vi "Dashboard Main.vi"() -> ()   [LabVIEW 2012]
uses:
  <vilib>/event_ctls.llb/eventvkey.ctl
  <vilib>/Utility/miscctls.llb/LVPointTypeDef.ctl
  <vilib>/Utility/config.llb/Read Key (String).vi
  <vilib>/Utility/config.llb/Read Key (I32).vi
  <vilib>/Utility/config.llb/Write Key (String).vi
  <vilib>/Utility/config.llb/Write Key (I32).vi
  <vilib>/Utility/config.llb/NI_LVConfig.lvlib
panel:
  in  "Camera Settings":T1={"Frate Rate"=30, "Compression"=70, "Size"=1} {"Frate Rate" scale=1.0..30.0; "Size" items=["640x480", "320x240", "160x120"]}
  out "Mode":T2(ring)=enum.""
  out "Camera IP":string="0.0.0.11"
  in  "Dashboard Tab":T3(tab)=enum."Drive Info"
  out "GO!! GO!! GO!!":bool
  out "Angle Ready":bool
  out "Shooter Speed":T4(ring)
  out "Shooter Encoder\nDead!!":bool
  out "Speed Ready":bool
  out "Dashboard Code Verzion":string
  out "Robot Code Version":string
  out "Display Loop speed (Hz)":dbl
  out "Shooter Angle":T5(ring)
  out "Shooter Good":bool
  out "Shooter Speed":dbl(graph)
  out "Wheel Speed":dbl
  out "Shooter Output":dbl
  out "Shooter Speed":T4(ring)
  out "Encoder Angle":dbl
  out "Debug Mode":bool
  out "Left Encoder":dbl
  out "Right Encoder":dbl
  out "Encoder Average":dbl
  out "Left Encoder Rate":dbl
  out "Right Encoder Rate":dbl
  out "Encoder Average Rate":dbl
  out "Gyro":dbl
  out "Battery Value":dbl(slide) scale=0.0..14.0 scale format="%#_2e"
  out "Battery":sgl(graph)
  out "JS1 Z":dbl(slide) scale=-1.0..1.0 scale format="%#_2e"
  out "JS2 Z":dbl(slide) scale=-1.0..1.0 scale format="%#_2e"
  out "Joystick 1":cluster{"X":dbl, "Y":dbl}[](graph)
  out "Joystick 2":cluster{"X":dbl, "Y":dbl}[](graph)
  out "JS Buttons 1":T6
  out "JS Buttons 2":T6
  out "MotorSlide4":dbl(slide) scale=-1.0..1.0 scale format="%#_2e"
  out "MotorSlide3":dbl(slide) scale=-1.0..1.0 scale format="%#_2e"
  out "MotorSlide2":dbl(slide) scale=-1.0..1.0 scale format="%#_2e"
  in  "MotorName3":string="Front Left"
  in  "MotorName4":string="Front Right"
  in  "MotorName1":string="Rear Left"
  in  "MotorName2":string="Rear Right"
  out "MotorChart4":dbl(graph)
  out "MotorChart3":dbl(graph)
  out "MotorChart2":dbl(graph)
  out "MotorSlide1":dbl(slide) scale=-1.0..1.0 scale format="%#_2e"
  out "MotorChart1":dbl(graph)
  out "Robot IP":string="0.0.0.0"
  in  "Debug Mode":bool
  in  "Slider":dbl(slide) scale=0.0..100.0 scale format="%#_3g"
  in  "On/Off":bool caption="Solenoid"
  in  "Test Name":u16(ring) items=["Select the test to run...", "Example Test", "-------------------------------", "List of tests is built in robot code.", "Replace with your own automated tests."]
  in  "Test Tree":string(tree)
  in  "Motor":cluster{"Value":dbl, "Enable":bool} {"Value" scale=-1.0..1.0 scale format="%#_3g"}
  out "Progress":T7 {"Test Progress" scale=0.0..100.0}
  in  "Rev/Fwd":cluster{"Forward":bool, "Reverse":bool}
  in  "Ring":u16(ring) items=["Auto", "Fixed indoor", "Fixed outdoor 1", "Fixed outdoor 2", "Fixed fluorescent 1", "Fixed fluorescent 2", "Hold current"]
  in  "Listbox":i32(listbox)
  in  "Viewer":T8(tab)
  in  "Enable Processing":bool
  out "Mbps":dbl format="%#.1g"
  in  "Enable":bool=TRUE
  in  "DB Camera Config":bool
  out "Mbps":bool
  out "fps":dbl format="%#.1g"
  out "Image Error Message":string="Timeout in Camera Communications"
  out "Camera Image":T9(plugin-control)
  out "Vision Angle":dbl
  out "Buttons 1":cluster{"1":bool, "2":bool, "3":bool}
  out "Kinect 1":cluster{"X":dbl, "Y":dbl, "Z":dbl} {"X" scale=1.0..-1.0; "Y" scale=1.0..-1.0; "Z" scale=1.0..-1.0}
  out "Buttons 2":cluster{"1":bool, "2":bool, "3":bool}
  out "Kinect 2":cluster{"X":dbl, "Y":dbl, "Z":dbl} {"X" scale=1.0..-1.0; "Y" scale=1.0..-1.0; "Z" scale=1.0..-1.0}
  out "Version":string
  out "Skeleton Picture":picture
  out "Players":i8
  out "Tree":string(tree)
  # "Drive & Motors"
  # "Robot IP:"
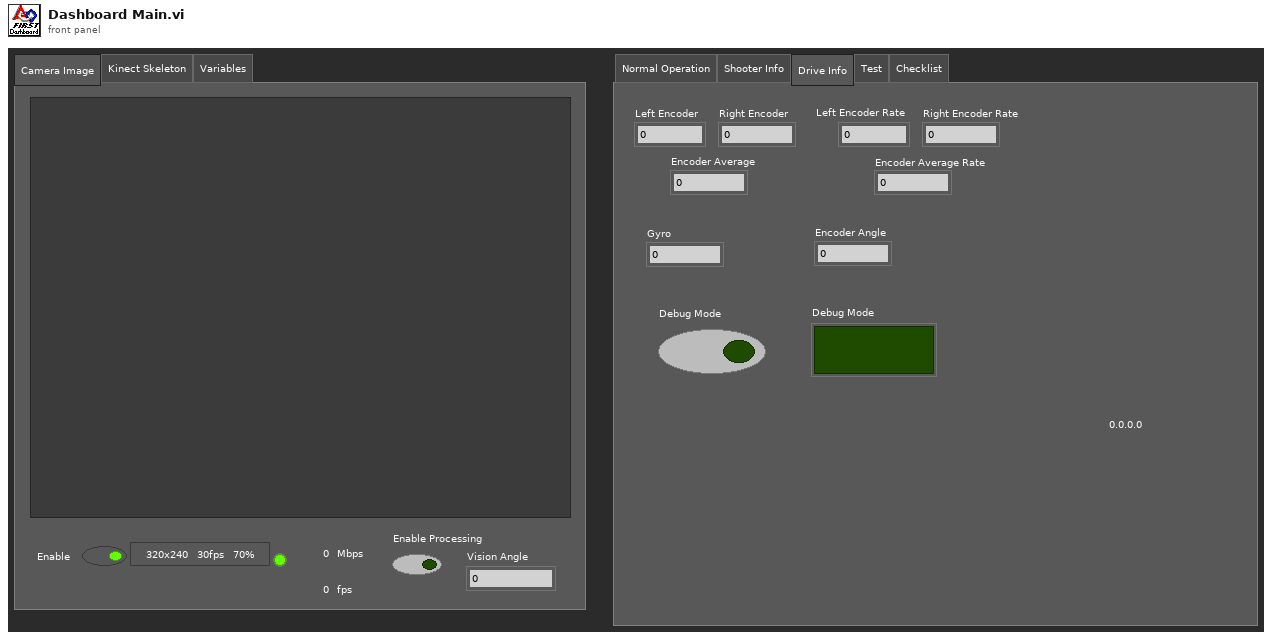
[diagram p1: front panel]
types:
  T1 = cluster{"Frate Rate":i32, "Compression":i32, "Size":u16}
  T2 = enum8{"Tele-Op Disabled", "Tele-Op Enabled", "Auto Disabled", "Auto Enabled", "Test Disabled", "Test Enabled", ""}
  T3 = enum32{"Normal Operation", "Shooter Info", "Drive Info", "Test", "Checklist"}
  T4 = enum16{"Off", "Close Pyramid 3pt", "Far Pyramid 3pt", "Feeder Shot", "UD Far 3pt Shot"}
  T5 = enum16{"Close 3pt Shot", "Far 3pt Shot", "Feeding"}
  T6 = cluster{bool, bool, bool, bool, bool, bool, bool, bool, bool, bool, bool, bool}
  T7 = cluster{"Test Progress":u8, "Test Progress Text":string}
  T8 = enum32{"Camera Image", "Kinect Skeleton", "Variables"}
  T9 = typedef "IMAQ Image.ctl" = refnum<image>
  T10 = typedef "Image Type" = u32
  T11 = cluster{"Competition mode":bool, "Robot Link":bool, "Autonomous":bool, "Enabled":bool, "E-Stop":bool, "Simulated":bool, "TestMode":bool, "Docked Window":bool}
  T12 = cluster{"Boolean Array[0]":bool, "Boolean Array[1]":bool, "Boolean Array[2]":bool, "Boolean Array[3]":bool, "Boolean Array[4]":bool, "Boolean Array[5]":bool, "Boolean Array[6]":bool, "Boolean Array[7]":bool, "Boolean Array[8]":bool, "Boolean Array[9]":bool, "Boolean Array[10]":bool, "Boolean Array[11]":bool}
  T13 = typedef "LVPointTypeDef.ctl" = cluster{"Horizontal":i16, "Vertical":i16}
  T14 = typedef "LVRectTypeDef.ctl" = cluster{"Left":i16, "Top":i16, "Right":i16, "Bottom":i16}
  T15 = typedef "LVBoundsTypeDef.ctl" = cluster{"Width":u32, "Height":u32}
  T16 = typedef "SkeletonTrackState.ctl" = enum32{"NotTracked", "PositionOnly", "Tracked"}
  T17 = cluster{"TrackingState":u8[], "Position":cluster{"x":sgl, "y":sgl, "z":sgl}, cluster{"x":sgl, "y":sgl, "z":sgl, sgl}[], "TrackState":T16}
  T18 = cluster{cluster{"ScaledToPercentRange":dbl, "ScaledToPercentRange":dbl, "ScaledToPercentRange":dbl}, cluster{bool, bool, bool}}[]
  T19 = cluster{cluster{"ScaledToPercentRange":dbl, "ScaledToPercentRange":dbl, "ScaledToPercentRange":dbl}, cluster{bool, bool, bool}}
  T20 = cluster{"ScaledToPercentRange":dbl, "ScaledToPercentRange":dbl, "ScaledToPercentRange":dbl}
  T21 = typedef "NI_LVConfig.lvlib/Config Data RefNum.ctl" = refnum<k1>
  T22 = typedef "eventvkey.ctl" = enum16{"ASCII", "Enter", "Return", "Shift", "Ctrl", "Alt", "Cmd", "Opt", "Caps", "NumLock", "Clear", "Break", "Up", "Down", "Left", "Right", "Insert", "Delete", "Home", "End", "PageUp", "PageDown", "Escape", "Help", "Pause", "ScrollLock", "F1", "F2", "F3", "F4", "F5", "F6", "F7", "F8", "F9", "F10", "F11", "F12", "F13", "F14", "F15", "F16", "F17", "F18", "F19", "F20", "F21", "F22", "F23", "F24", "Play", "VolumeUp", "VolumeDown", "Mute", "Two Byte Char"}
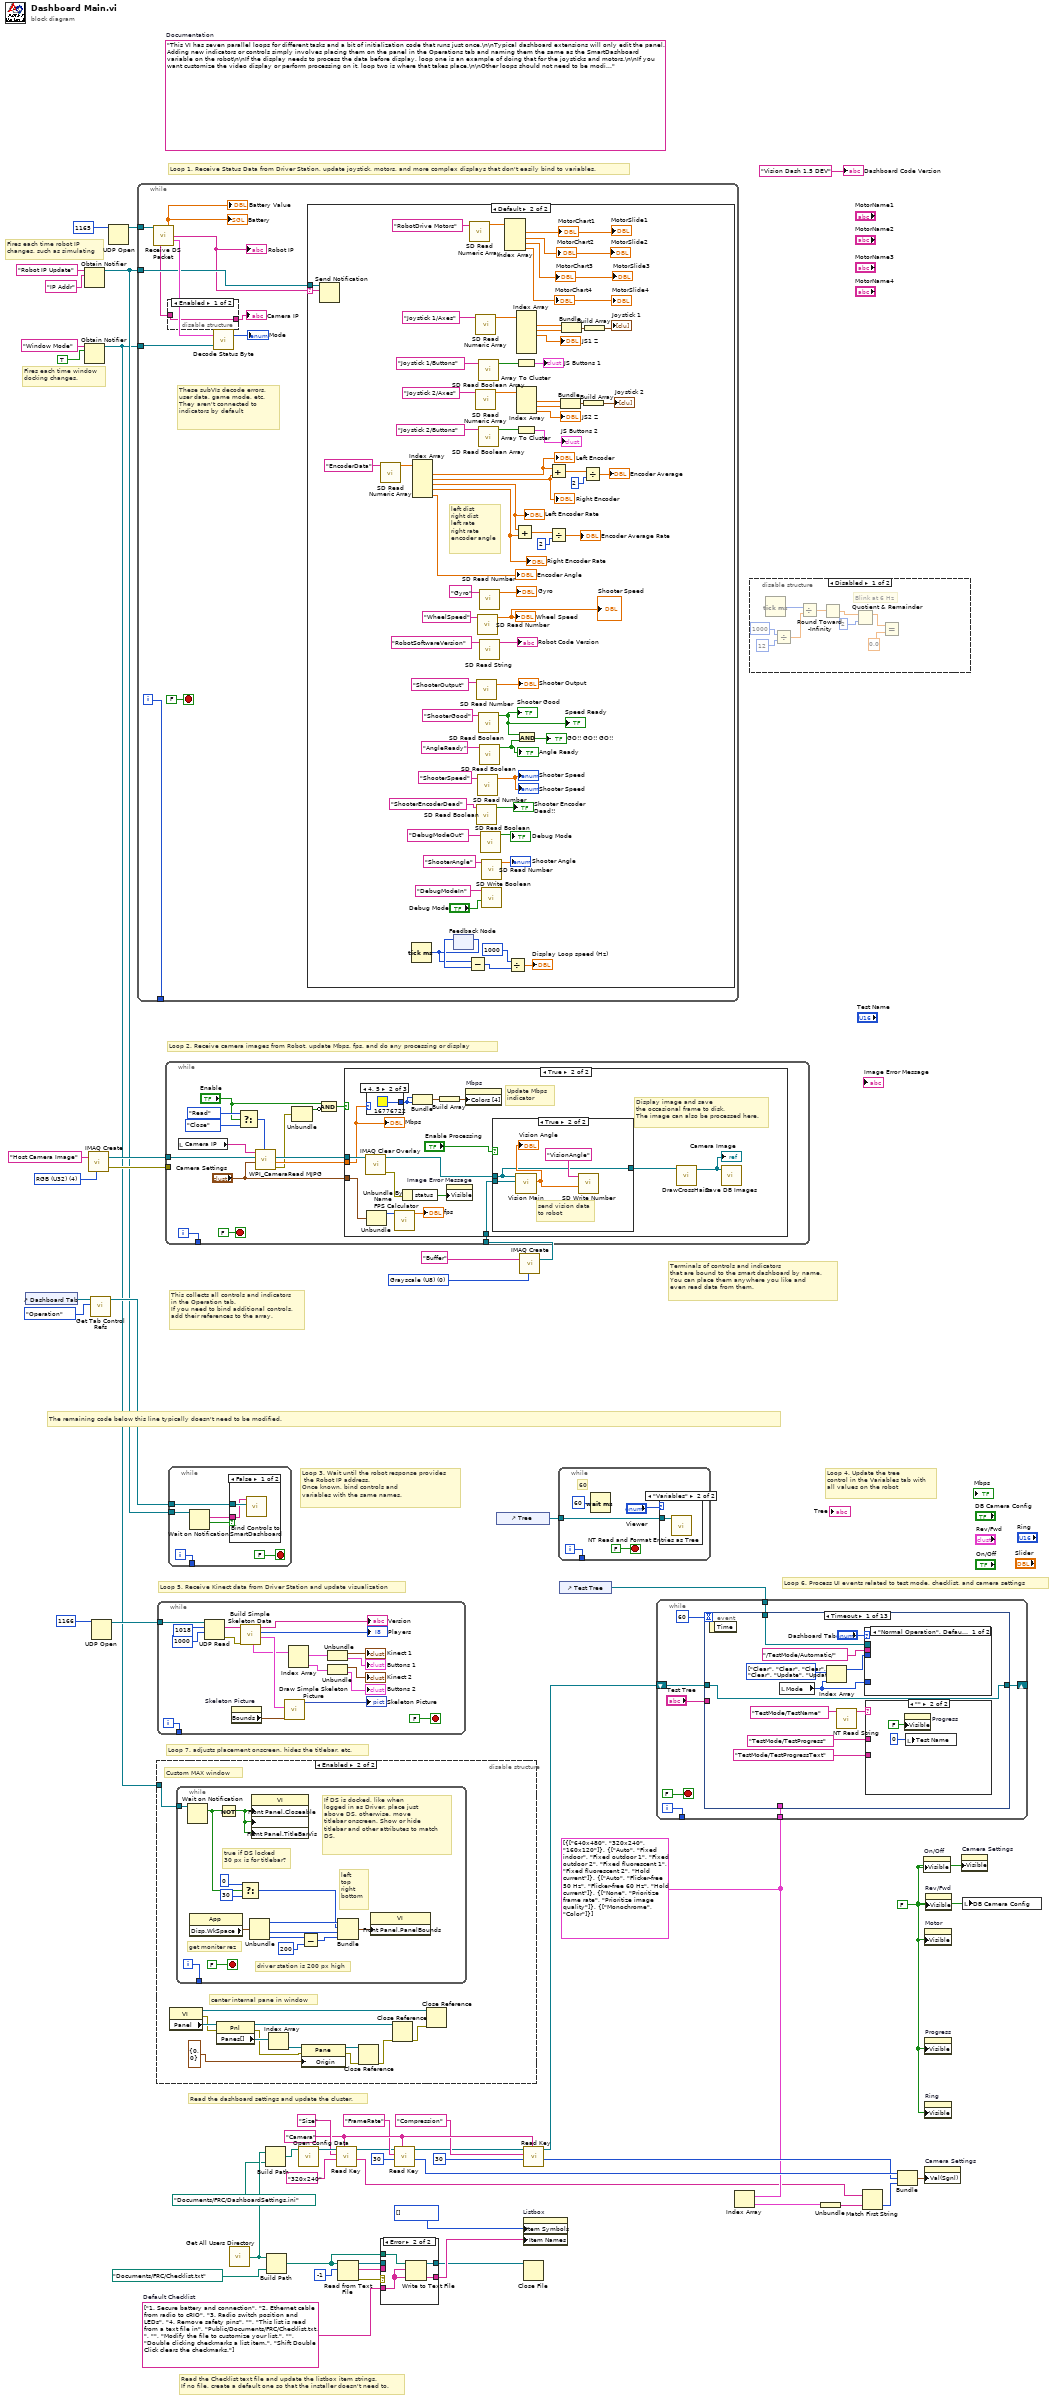
[diagram p0: block diagram]
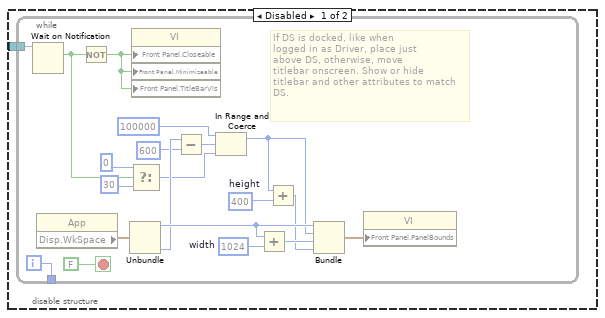
[diagram p3: hidden frame]
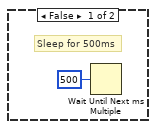
[diagram p5: hidden frame]
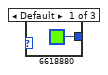
[diagram p7: hidden frame]
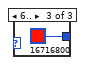
[diagram p8: hidden frame]
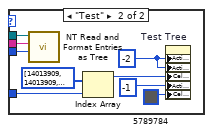
[diagram p10: hidden frame]
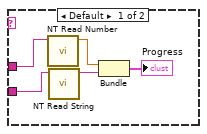
[diagram p11: hidden frame]
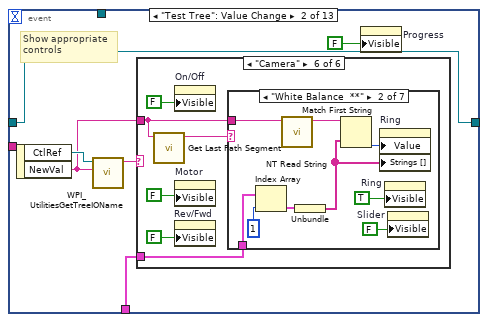
[diagram p12: hidden frame]
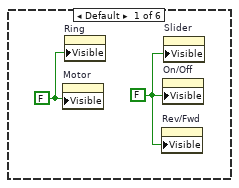
[diagram p13: hidden frame]
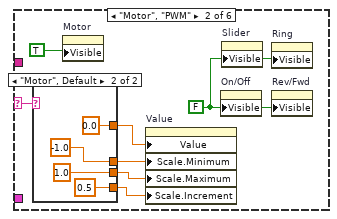
[diagram p14: hidden frame]
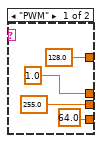
[diagram p15: hidden frame]
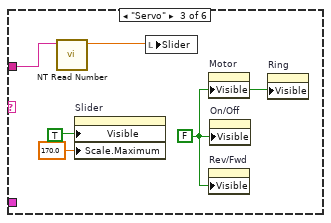
[diagram p16: hidden frame]
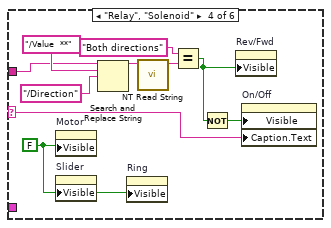
[diagram p17: hidden frame]
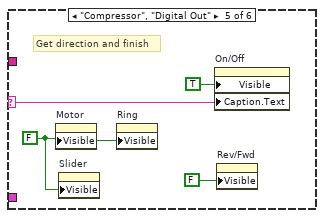
[diagram p18: hidden frame]
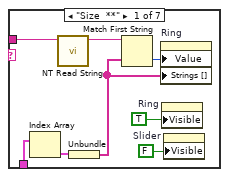
[diagram p19: hidden frame]
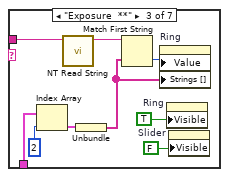
[diagram p20: hidden frame]
diagram:
  w3 = T10 0 items=["Grayscale (U8)", "Grayscale (I16)", "Grayscale (SGL)", "Complex (CSG)", "RGB (U32)", "HSL (U32)", "RGB (U64)", "Grayscale (U16)"] ("Image Type")
  w25 = "Camera"
  w17 = cluster{string[]}[] [{["640x480", "320x240", "160x120"]}, {["Auto", "Fixed indoor", "Fixed outdoor 1", "Fixed outdoor 2", "Fixed fluorescent 1", "Fixed fluorescent 2", "Hold current"]}, {["Auto", "Flicker-free 50 Hz", "Flicker-free 60 Hz", "Hold current"]}, {["None", "Prioritize frame rate", "Prioritize image quality"]}, {["Monochrome", "Color"]}]
  w33 = string[] ["1. Secure battery and connection", "2. Ethernet cable from radio to cRIO", "3. Radio switch position and LEDs", "4. Remove safety pins", "", "This list is read from a text file in", "Public/Documents/FRC/Checklist.txt.", "", "Modify the file to customize your list.", "", "Double clicking checkmarks a list item.", "Shift Double Click clears the checkmarks."]  # Default Checklist
  w31 = FALSE ("Visible")
  (unwired) "This VI has seven parallel loops for different tasks and a bit of initialization code that runs just once.\n\nTypical dashboard extensions will only edit the panel. Adding new indicators or controls simply involves placing them on the panel in the Operations tab and naming them the same as the SmartDashboard variable on the robot\n\nIf the display needs to process the data before display, loop one is an example of doing that for the joysticks and motors.\n\nIf you want customize the video display or perform processing on it, loop two is where that takes place.\n\nOther loops should not need to be modified. They are pretty standard, and document the task they perform."  # Documentation
  w54 = T10 4 items=["Grayscale (U8)", "Grayscale (I16)", "Grayscale (SGL)", "Complex (CSG)", "RGB (U32)", "HSL (U32)", "RGB (U64)"] ("Image Type")
  # "Fires each time robot IP\nchanges, such as simulating"
  # "Fires each time window\ndocking changes."
  # "Read the Checklist text file and update the listbox item strings.\nIf no file, create a default one so that the installer doesn't need to."
  # "This collects all controls and indicators\nin the Operation tab.\nIf you need to bind additional controls,\nadd their references to the array."
  # "The remaining code below this line typically doesn't need to be modified."
  # "Loop 6. Process UI events related to test mode, checklist, and camera settings"
  # "Read the dashboard settings and update the cluster."
  # "Terminals of controls and indicators\nthat are bound to the smart dashboard by name.\nYou can place them anywhere you like and\neven read data from them."
  # "Loop 4. Update the tree\ncontrol in the Variables tab with\nall values on the robot"
  # "Loop 3. Wait until the robot response provides\n the Robot IP address.\nOnce known, bind controls and\nvariables with the same names."
  # "Loop 5. Receive Kinect data from Driver Station and update visualization"
  # "Loop 7. adjusts placement onscreen, hides the titlebar, etc."
  # "Loop 1. Receive Status Data from Driver Station, update joystick, motors, and more complex displays that don't easily bind to variables."
  # "Loop 2. Receive camera images from Robot, update Mbps, fps, and do any processing or display"
  n1 = control-ref of="Dashboard Tab"() -> (w47:refnum<vi>)
  n2 = Obtain Notifier(name (unnamed)="Robot IP Update", notification data type="IP Addr" ("name (unnamed)")) -> (notifier out=w44:refnum<notifier>)  [unwired: 2 in, 2 out]
  n3 = Obtain Notifier(name (unnamed)="Window Mode", notification data type=TRUE) -> (notifier out=w37:refnum<notifier>)  [unwired: 2 in, 2 out]
  n4 = call "IMAQ Create"("Image Name"="Host Camera Image", "Image Type"=w54) -> ("New Image"=w52:T9, "error out"=w51:errorcluster)  [unwired: 2 in, 1 out]
  n5 = call <vilib>:"Get Tab Control Refs.vi"("Page Index"=enum32{"Operation", "Test"}."Operation" ("Dashboard Tab"), "TabControl in"=w47) -> ("ControlsOnPage"=w48:refnum<vi>[])  [unwired: 9 in]
  n6 = UDP Open(11:u16 1166 ("port")) -> (port=w49:refnum<k16>)  [unwired: 2 in, 4 out]
  n7 = UDP Open(11:u16 1165 ("port")) -> (port=w55:refnum<k16>)  [unwired: 2 in, 4 out]
  n8 = while {
    tunnel: w55 -> [w65]
    tunnel: w44 -> [w60]
    tunnel: w37 -> [w63]
    tunnel: [w61] -> _
    i -> [w61]
    stop <- FALSE stop-if-true
    # "These subVIs decode errors, user data, game mode, etc.\nThey aren't connected to indicators by default"
    n9 = call "Receive DS Packet.vi"("Recv Socket"=w65) -> ("Battery"=→"Battery" →"Battery Value":sgl, "Robot IP Address"=w59:string, "Status"=w66:T11, "Camera IP Address"=w57:string)  [unwired: 1 in, 10 out]
    "Robot IP" <- w59
    n10 = disable-structure shown="Enabled" {
      disable-tunnel: [w68 "10.16.76.11" ("Camera IP")] -> w58
      disable-tunnel: w57 -> [w68 _]
      frame Enabled {
      }
      frame Disabled {
      }
    }
    "Camera IP" <- w58
    n11 = call "Decode Status Byte.vi"("Window Mode Notifier"=w63, "Status"=w66) -> ("Mode"=→"Mode":T2)  [unwired: 1 out]
    n12 = case shown="Default" w59 {
      selector: w59 -> [_ w111]
      tunnel: w60 -> [_ w112]
      frame "0.0.0.0" {
        # "Robot not responding, don't poll the variables"
      }
      frame Default {
        # "left dist\nright dist\nleft rate\nright rate\nencoder angle"
        n13 = Send Notification(notification=w111, notifier=w112) -> ()  [unwired: 1 in, 2 out]
        n14 = call <vilib>:"SD Read Numeric Array.vi"("Name"="EncoderData") -> ("Numeric Array"=w98:dbl[])  [unwired: 8 in, 2 out]
        n15 = Tick Count (ms)() -> (millisecond timer value=w80:u32)
        n16 = Index Array(array=w98) -> (element #1=w97:dbl, element #2=w96:dbl, element #3=w92:dbl, element #4=w91:dbl, element #5=→"Encoder Angle":dbl)  [unwired: 5 in]
        "Left Encoder" <- w97
        "Right Encoder" <- w96
        "Left Encoder Rate" <- w92
        "Right Encoder Rate" <- w91
        n17 = feedback-in #1(w80) -> ()
        n18 = feedback #1() -> (w81:u32)  [unwired: 1 in]
        n19 = Subtract(x=w80, y=w81) -> (x-y=w79:u32)
        n20 = call <vilib>:"SD Read Numeric Array.vi"("Name"="RobotDrive Motors") -> ("Numeric Array"=w135:dbl[])  [unwired: 8 in, 2 out]
        n21 = call <vilib>:"SD Read Numeric Array.vi"("Name"="Joystick 1/Axes") -> ("Numeric Array"=w128:dbl[])  [unwired: 8 in, 2 out]
        n22 = call <vilib>:"SD Read Numeric Array.vi"("Name"="Joystick 2/Axes") -> ("Numeric Array"=w122:dbl[])  [unwired: 8 in, 2 out]
        n23 = call <vilib>:"SD Read Number.vi"("Name"="ShooterOutput") -> ("Numeric"=→"Shooter Output":dbl)  [unwired: 8 in, 2 out]
        n24 = call <vilib>:"SD Read Boolean.vi"("Name"="ShooterEncoderDead") -> ("Boolean"=→"Shooter Encoder\nDead!!":bool)  [unwired: 8 in, 2 out]
        n25 = call <vilib>:"SD Read Number.vi"("Name"="ShooterSpeed") -> ("Numeric"=→"Shooter Speed" →"Shooter Speed":dbl)  [unwired: 8 in, 2 out]
        n26 = call <vilib>:"SD Read Number.vi"("Name"="WheelSpeed") -> ("Numeric"=→"Wheel Speed" →"Shooter Speed":dbl)  [unwired: 8 in, 2 out]
        n27 = call <vilib>:"SD Read Boolean Array.vi"("Name"="Joystick 1/Buttons") -> ("Boolean Array"=w130:bool[])  [unwired: 8 in, 2 out]
        n28 = call <vilib>:"SD Read Boolean Array.vi"("Name"="Joystick 2/Buttons") -> ("Boolean Array"=w121:bool[])  [unwired: 8 in, 2 out]
        n29 = call <vilib>:"SD Read Boolean.vi"("Name"="ShooterGood") -> ("Boolean"=w85:bool)  [unwired: 8 in, 2 out]
        "Shooter Good" <- w85
        "Speed Ready" <- w85
        n30 = call <vilib>:"SD Read Number.vi"("Name"="Gyro") -> ("Numeric"=→"Gyro":dbl)  [unwired: 8 in, 2 out]
        n31 = call <vilib>:"SD Read String.vi"("Name"="RobotSoftwareVersion") -> ("String"=→"Robot Code Version":string)  [unwired: 8 in, 2 out]
        n32 = call <vilib>:"SD Read Boolean.vi"("Name"="AngleReady") -> ("Boolean"=w84:bool)  [unwired: 8 in, 2 out]
        "Angle Ready" <- w84
        n33 = call <vilib>:"SD Read Boolean.vi"("Name"="DebugModeOut") -> ("Boolean"=→"Debug Mode":bool)  [unwired: 8 in, 2 out]
        n34 = call <vilib>:"SD Read Number.vi"("Name"="ShooterAngle") -> ("Numeric"=→"Shooter Angle":dbl)  [unwired: 8 in, 2 out]
        n35 = call <vilib>:"SD Write Boolean.vi"("Boolean"="Debug Mode", "Name"="DebugModeIn") -> ()  [unwired: 8 in, 2 out]
        n36 = Index Array(array=w135) -> (element #1=→"MotorChart1" →"MotorSlide1":dbl, element #2=→"MotorSlide2" →"MotorChart2":dbl, element #3=→"MotorChart3" →"MotorSlide3":dbl, element #4=→"MotorChart4" →"MotorSlide4":dbl)  [unwired: 4 in]
        n37 = Divide(x=1000, y=w79) -> (x/y=→"Display Loop speed (Hz)":dbl)
        n38 = Add(x=w92, y=w91) -> (x+y=w93:dbl)
        n39 = Array To Cluster(array=w130) -> (cluster=→"JS Buttons 1":T12)
        n40 = Array To Cluster(array=w121) -> (cluster=→"JS Buttons 2":T12)
        n41 = Index Array(array=w128) -> (element #1=w125:dbl, element #2=w126:dbl, element #3=→"JS1 Z":dbl)  [unwired: 6 in, 3 out]
        n42 = Index Array(array=w122) -> (element #1=w117:dbl, element #2=w116:dbl, element #3=→"JS2 Z":dbl)  [unwired: 3 in]
        n43 = And(x=w85, y=w84) -> (x .and. y?=→"GO!! GO!! GO!!":bool)
        n44 = Add(x=w97, y=w96) -> (x+y=w107:dbl)
        n45 = Divide(x=w93, y=2) -> (x/y=→"Encoder Average Rate":dbl)
        n46 = Bundle("Numeric"=w117, "Numeric"=w116) -> (w118:cluster{"Numeric":dbl, "Numeric":dbl})  [unwired: 1 in]
        n47 = Bundle("Numeric"=w125, "Numeric"=w126) -> (w124:cluster{"Numeric":dbl, "Numeric":dbl})  [unwired: 1 in]
        n48 = Divide(x=w107, y=2) -> (x/y=→"Encoder Average":dbl)
        n49 = Build Array(w118) -> (→"Joystick 2":cluster{"Numeric":dbl, "Numeric":dbl}[])
        n50 = Build Array(w124) -> (→"Joystick 1":cluster{"Numeric":dbl, "Numeric":dbl}[])
      }
    }
  }
  n51 = disable-structure shown="Enabled" {
    disable-tunnel: w37 -> [w139 w172]
    frame Disabled {
      n52 = while {
        tunnel: w139 -> [w158]
        tunnel: [w156] -> _
        i -> [w156]
        stop <- FALSE stop-if-true
        w148 = 1024  # width
        w151 = 400  # height
        # "If DS is docked, like when\nlogged in as Driver, place just\nabove DS, otherwise, move\ntitlebar onscreen. Show or hide\ntitlebar and other attributes to match\nDS."
        n53 = Wait on Notification(notifier=w158) -> (notification=w143:bool)  [unwired: 3 in, 3 out]
        n54 = property class="App"() -> ("Disp.WkSpace"=w154:T14)  [unwired: 2 in, 2 out]
        n55 = Not(x=w143) -> (.not. x?=w157:bool)
        n56 = Unbundle(w154) -> ("Left"=w152:i16, "Bottom"=w149:i16)  [unwired: 2 out]
        n57 = Select(t=0, s=w143, f=30) -> (s? t:f=w142:i32)
        n58 = property class="VI"("Front Panel.Closeable"=w157, "Front Panel.Minimizeable"=w157, "Front Panel.TitleBarVis"=w157) -> ()  [unwired: 2 in, 2 out]
        n59 = Subtract(x=w149, y=600) -> (x-y=w146:i32)
        n60 = In Range and Coerce(upper limit=100000, x=w146, lower limit=w142) -> (coerced(x)=w140:i32)  [unwired: 1 out]
        n61 = Add(x=w152, y=w148) -> (x+y=w153:i32)
        n62 = Add(x=w140, y=w151) -> (x+y=w150:i32)
        n63 = Bundle("Left"=w152, w140, w153, w150) -> (w155:cluster{"Left":i16, i32, i32, i32})  [unwired: 1 out]
        n64 = property class="VI"("Front Panel.PanelBounds"=w155) -> ()  [unwired: 2 in, 2 out]
      }
    }
    frame Enabled {
      # "center internal pane in window"
      # "Custom MAX window"
      n65 = property class="VI"() -> (reference out=w165:refnum<vi>, error out=w164:errorcluster, "Panel"=w171:refnum<vi>)  [unwired: 2 in]
      n66 = while {
        tunnel: w172 -> [w186]
        tunnel: [w184] -> _
        i -> [w184]
        stop <- FALSE stop-if-true
        # "driver station is 200 px high"
        # "true if DS locked\n30 px is for titlebar?"
        # "left\ntop\nright\nbottom"
        # "get moniter rez"
        # "If DS is docked, like when\nlogged in as Driver, place just\nabove DS, otherwise, move\ntitlebar onscreen. Show or hide\ntitlebar and other attributes to match\nDS."
        n67 = Wait on Notification(notifier=w186) -> (notification=w178:bool)  [unwired: 3 in, 3 out]
        n68 = property class="App"() -> ("Disp.WkSpace"=w182:T14)  [unwired: 2 in, 2 out]
        n69 = Not(x=w178) -> (.not. x?=w185:bool)
        n70 = Select(t=0, s=w178, f=30) -> (s? t:f=w176:i32)
        n71 = Unbundle(w182) -> ("Left"=w181:i16, "Right"=w177:i16, "Bottom"=w174:i16)  [unwired: 1 out]
        n72 = property class="VI"("Front Panel.Closeable"=w185, "Front Panel.Minimizeable"=w185, "Front Panel.TitleBarVis"=w185) -> ()  [unwired: 2 in, 2 out]
        n73 = Subtract(x=w174, y=i16 200) -> (x-y=w175:i16)
        n74 = Bundle("Left"=w181, w176, "Right"=w177, w175) -> (w183:cluster{"Left":i16, i32, "Right":i16, i16})  [unwired: 1 out]
        n75 = property class="VI"("Front Panel.PanelBounds"=w183) -> ()  [unwired: 2 in, 2 out]
      }
      n76 = property class="Pnl"(reference=w171, error in=w164) -> (reference out=w166:refnum<vi>, error out=w163:errorcluster, "Panes[]"=w170:refnum<vi>[])
      n77 = Index Array(array=w170) -> (element=w169:refnum<vi>)  [unwired: 1 in]
      n78 = property class="Pane"(reference=w169, error in=w163, "Origin"=T13 {"Horizontal"=0, "Vertical"=0}) -> (reference out=w167:refnum<vi>, error out=w162:errorcluster)
      n79 = Close Reference(reference=w167, error in (no error)=w162) -> (error out=w161:errorcluster)
      n80 = Close Reference(reference=w166, error in (no error)=w161) -> (error out=w160:errorcluster)
      n81 = Close Reference(reference=w165, error in (no error)=w160) -> ()  [unwired: 1 out]
    }
  }
  n82 = while {
    tunnel: w49 -> [w204]
    tunnel: [w189] -> _
    i -> [w189]
    stop <- FALSE stop-if-true
    n83 = UDP Read(connection ID=w204, max size (548)=1018 ("bytes to read"), timeout ms (25000)=1000) -> (data out=w198:string, error out=w188:errorcluster)  [unwired: 1 in, 3 out]
    n84 = property on="Skeleton Picture" class="Pict"() -> ("Bounds"=w200:T15)  [unwired: 2 in, 2 out]
    n85 = call "Build Simple Skeleton Data.vi"("error in (no error)"=w188, "data in"=w198) -> ("Skeleton Data"=w199:T17, "NumPlayers"=→"Players":i8, "Version String"=→"Version":string, "Simple Joystick Info"=w196:T18)  [unwired: 5 in, 1 out]
    n86 = call "Draw Simple Skeleton Picture.vi"("Bounds"=w200, "Simple Skeleton"=w199) -> ("new picture out"=→"Skeleton Picture":picture)  [unwired: 9 in]
    n87 = Index Array(array=w196) -> (element #1=w195:T19, element #2=w194:T19)  [unwired: 2 in]
    n88 = Unbundle(w195) -> (→"Kinect 1":T20, →"Buttons 1":cluster{bool, bool, bool})
    n89 = Unbundle(w194) -> (→"Kinect 2":T20, →"Buttons 2":cluster{bool, bool, bool})
  }
  n90 = while {
    tunnel: w48 -> [w212]
    tunnel: w44 -> [w209]
    tunnel: [w207] -> _
    i -> [w207]
    stop <- FALSE stop-if-true
    n91 = Wait on Notification(notifier=w209) -> (notification=w208:string, timed out?=w210:bool)  [unwired: 3 in, 2 out]
    n92 = case shown="False" w210 {
      tunnel: w212 -> [w214 _]
      tunnel: w208 -> [w213 _]
      frame False {
        n93 = call <vilib>:"Bind Controls to SmartDashboard.vi"("Bound Control Refs"=w214, "Server IP Address"=w213) -> ()  [unwired: 10 in]
      }
      frame True {
      }
    }
  }
  n94 = call "Get All Users Directory.vi"() -> ("All User Path"=w30:path)
  n95 = Build Path(base path=w30, name or relative path=path "Documents/FRC/DashboardSettings.ini") -> (appended path=w29:path)
  n96 = Build Path(base path=w30, name or relative path=path "Documents/FRC/Checklist.txt") -> (appended path=w34:path)
  n97 = call <vilib>:"Open Config Data.vi"("configuration file path"=w29) -> ("refnum"=w28:T21)  [unwired: 8 in, 2 out]
  n98 = call-poly <vilib>:"Read Key.vi"("section"=w25, "default value"="320x240", "key"="Size", "refnum"=w28) -> ("value"=w15:string, "refnum out"=w10:T21)  [unwired: 2 in, 4 out]
  n99 = Read from Text File(file (use dialog)=w34, count=-1 ("timeout ms (25000)")) -> (refnum out=w12:refnum<file>, text=w35:string[], error out=w36:errorcluster)  [unwired: 2 in, 1 out]
  n100 = case shown="Error" w36 {
    tunnel: w35 -> [w216 _]
    tunnel: [w216 w218] -> w32
    tunnel: w33 -> [_ w218]
    tunnel: w34 -> [_ w219]
    tunnel: [w215 w217] -> w11
    tunnel: w12 -> [w215 _]
    frame No Error {
    }
    frame Error {
      n101 = Write to Text File(file (use dialog)=w219, text=w218) -> (refnum out=w217:refnum<file>)  [unwired: 2 in, 2 out]
    }
  }
  n102 = call-poly <vilib>:"Read Key.vi"("section"=w25, "default value"=30, "key"="FrameRate", "refnum"=w10) -> ("value"=w20:i32, "refnum out"=w9:T21)  [unwired: 1 in, 5 out]
  n103 = control-ref of="Tree"() -> (w6:refnum<vi>)
  n104 = call "IMAQ Create"("Image Name"="Buffer", "Image Type"=w3) -> ("New Image"=w2:T9)  [unwired: 3 in, 1 out]
  n105 = while {
    tunnel: w52 -> [w230]
    tunnel: w51 -> [_]
    tunnel: [w233] -> _
    tunnel: w2 -> [w220]
    i -> [w233]
    stop <- FALSE stop-if-true
    n106 = local read "Camera IP"() -> (w232:string)
    n107 = Select(t=enum16{"Read", "Reopen", "Close"}."Read" ("Operation"), s="Enable", f=enum16{"Read", "Reopen", "Close"}."Close" ("Operation")) -> (s? t:f=w225:enum16{"Read", "Reopen", "Close"})
    n108 = call <vilib>:"WPI_CameraRead MJPG.vi"("Operation"=w225, "Camera Settings"="Camera Settings", "Image"=w230, "address"=w232) -> ("error out"=w224:errorcluster, "Bandwidth (kbps)"=w228:dbl, "Image Out"=w229:T9)  [unwired: 5 in]
    n109 = Unbundle(w224) -> ("status"=w222:bool)  [unwired: 2 out]
    n110 = Compound Arithmetic op=AND("Enable", invert w222) -> (w221:bool)
    n111 = case shown="True" w221 {
      tunnel: "Camera Settings" -> [_ w242]
      tunnel: w229 -> [_ w245]
      tunnel: w228 -> [_ w244]
      tunnel: w220 -> [_ w240]
      frame False {
        # "Sleep for 500ms"
        n112 = Wait Until Next ms Multiple(millisecond multiple=u32 500) -> ()  [unwired: 1 out]
      }
      frame True {
        # "Display image and save\nthe occasional frame to disk.\nThe image can also be processed here."
        # "Update Mbps\nindicator"
        n113 = call "IMAQ Clear Overlay"("Image"=w245) -> ("error out"=w249:errorcluster, "Image Out"=w238:T9)  [unwired: 2 in, 7 out]
        n114 = case shown="4, 5" w244 {
          tunnel: [u32 6618880 ("Color Box") u32 16776722 ("Color Box") u32 16716800 ("Color Box")] -> w246
          frame Default {
          }
          frame 4, 5 {
          }
          frame 6.. {
          }
        }
        n115 = Unbundle(w242) -> ("Frate Rate"=w241:i32)  [unwired: 2 out]
        n116 = call "FPS Calculator.vi"("Average Count"=w241) -> ("fps"=→"fps":dbl)  [unwired: 10 in]
        n117 = Unbundle By Name(w249) -> ("status"=w250:bool)
        n118 = Bundle("Color Box"=w246, "Color Box"=w246) -> (w248:cluster{"Color Box":u32, "Color Box":u32})  [unwired: 1 out]
        n119 = Build Array(w248) -> (w247:cluster{"Color Box":u32, "Color Box":u32}[])
        n120 = property on="Image Error Message" class="Str"("Visible"=w250) -> ()  [unwired: 2 in, 2 out]
        n121 = property on="Mbps" class="Bool (strict)"("Colors [4]"=w247) -> ()  [unwired: 2 in, 2 out]
        n122 = case shown="True" "Enable Processing" {
          tunnel: w240 -> [_ w255]
          tunnel: w238 -> [w251 w252]
          tunnel: [w251 w252] -> w237
          frame False {
          }
          frame True {
            # "send vision data\nto robot"
            n123 = call "Vision Main.vi"("Frame Buffer"=w255, "Camera Image"=w252) -> ("Chosen Target Angle"=w253:dbl)  [unwired: 8 in, 1 out]
            "Vision Angle" <- w253
            n124 = call <vilib>:"SD Write Number.vi"("Numeric"=w253, "Name"="VisionAngle") -> ()  [unwired: 8 in, 2 out]
          }
        }
        n125 = call "DrawCrossHairs.vi"("Image In"=w237) -> ("Image Out"=w239:T9)  [unwired: 10 in]
        "Camera Image" <- w239
        n126 = call "Save DB Images.vi"("Image"=w239) -> ()  [unwired: 2 in, 1 out]
        "Mbps" <- w244
      }
    }
  }
  n127 = property on="Listbox" class="LstBox (strict)"("Item Symbols"=i32[] [], "Item Names"=w32) -> ()  [unwired: 2 in, 2 out]
  n128 = Close File(refnum=w11) -> ()  [unwired: 1 in, 2 out]
  n129 = call-poly <vilib>:"Read Key.vi"("section"=w25, "default value"=30, "key"="Compression", "refnum"=w9) -> ("value"=w19:i32, "refnum out"=w7:T21)  [unwired: 1 in, 5 out]
  n130 = while {
    tunnel: [w260] -> _
    tunnel: w6 -> [w259]
    i -> [w260]
    stop <- FALSE stop-if-true
    # "60"
    n131 = Wait (ms)(milliseconds to wait=u32 60) -> ()  [unwired: 1 out]
    n132 = case shown="\"Variables\"" "Viewer" {
      tunnel: w259 -> [_ w264]
      frame Default {
      }
      frame "Variables" {
        n133 = call <vilib>:"NT Read and Format Entries as Tree.vi"("Tree Refnum"=w264) -> ()  [unwired: 9 in, 2 out]
      }
    }
  }
  n134 = control-ref of="Test Tree"() -> (w5:refnum<vi>)
  n135 = while {
    tunnel: w17 -> [w269]
    shift-right: [w268] -> _
    shift-left: w7 -> [w267]
    tunnel: [w266] -> _
    tunnel: w5 -> [w265]
    i -> [w266]
    stop <- FALSE stop-if-true
    n136 = event shown="[0] Timeout" {
      selector: _ -> [_ _ _ _ _ _ _ _ _ _ _ _ _]
      dyn-events: _ -> [_ _ _ _ _ _ _ _ _ _ _ _ _]
      timeout: u32 60 ("milliseconds to wait") -> [_ _ _ _ _ _ _ _ _ _ _ _ _]
      tunnel: w265 -> [w279 _ _ _ _ _ _ _ _ _ _ _ _]
      tunnel: "Test Tree" -> [_ _ _ _ _ _ _ _ w473 w481 w483 w487 w495]
      tunnel: w269 -> [_ w301 _ _ _ _ w437 w467 _ _ _ _ _]
      tunnel: [w273 w300 _ w403 w411 w423 w436 w460 w472 w479 w482 w486 w494] -> w268
      tunnel: w267 -> [w273 w300 _ w403 w411 w423 w435 w460 w472 w479 w482 w486 w494]
      event Timeout {
        w278 = enum16{"Update", "Clear"}[] [enum."Clear", enum."Clear", enum."Clear", enum."Clear", enum."Update", enum."Update", enum."Clear"] items=["Update", "Clear"]
        n137 = event-data() -> ()  [unwired: 1 in, 1 out]
        n138 = local read "Mode"() -> (w276:T2)
        n139 = Index Array(array=w278, index=w276) -> (element=w277:enum16{"Update", "Clear"})
        n140 = call <vilib>:"NT Read String.vi"("Name"="TestMode/TestName") -> ("String"=w282:string)  [unwired: 9 in, 1 out]
        n141 = case shown="\"Normal Operation\", Default" "Dashboard Tab" {
          tunnel: w279 -> [_ w292]
          tunnel: "/TestMode/Automatic/" ("Name Pattern") -> [_ w291]
          tunnel: w277 -> [_ w290]
          tunnel: w276 -> [_ w288]
          frame "Normal Operation", Default {
          }
          frame "Test" {
            w287 = -2 ("Active Item:Row Number")
            n142 = call <vilib>:"NT Read and Format Entries as Tree.vi"("Operation"=w290, "Name Pattern"=w291, "Tree Refnum"=w292) -> ()  [unwired: 7 in, 2 out]
            n143 = Index Array(array=u32[] [14013909, 14013909, 14013909, 14013909, 14013909, 16777215, 14013909], index=w288) -> (element=w286:u32)
            n144 = property on="Test Tree" class="Tree (strict)"("Active Item Row Number"=w287, "ActiveColNum"=w287, "CellBG"=w286, "Active Item Row Number"=-1 ("Active Item:Row Number"), "CellBG"=u32 5789784 ("Color Box")) -> ()  [unwired: 2 in, 2 out]
          }
        }
        n145 = case shown="\"\"" w282 {
          tunnel: "TestMode/TestProgress" ("Name") -> [w294 _]
          tunnel: "TestMode/TestProgressText" ("Name") -> [w293 _]
          frame Default {
            n146 = call <vilib>:"NT Read Number.vi"("Name"=w294) -> ("Numeric"=w295:dbl)  [unwired: 9 in, 1 out]
            n147 = call <vilib>:"NT Read String.vi"("Name"=w293) -> ("String"=w296:string)  [unwired: 9 in, 1 out]
            n148 = Bundle("Numeric"=w295, "String"=w296) -> (→"Progress":cluster{"Numeric":dbl, "String":string})  [unwired: 1 in]
          }
          frame "" {
            n149 = property on="Progress" class="Clust (strict)"("Visible"=FALSE) -> ()  [unwired: 2 in, 2 out]
            n150 = local write "Test Name"(u16 0) -> ()
          }
        }
      }
      event "Test Tree": Value Change {
        # "Show appropriate\ncontrols"
        n151 = event-data() -> ("CtlRef"=w304:refnum<vi>, "NewVal"=w302:string)  [unwired: 1 in]
        n152 = call <vilib>:"WPI_UtilitiesGetTreeIOName.vi"("NewVal"=w302, "TreeControl in"=w304) -> ("I/O Name"=w305:string)  [unwired: 9 in]
        n153 = case shown="\"Camera\"" w305 {
          selector: w305 -> [_ w312 _ w330 w339 _]
          tunnel: w302 -> [_ _ w327 w329 _ w346]
          tunnel: w301 -> [_ _ _ _ _ w345]
          frame Default {
            w307 = FALSE ("Visible")
            w306 = FALSE ("Visible")
            n154 = property on="Motor" class="Clust (strict)"("Visible"=w306) -> ()  [unwired: 2 in, 2 out]
            n155 = property on="Ring" class="Ring (strict)"("Visible"=w306) -> ()  [unwired: 2 in, 2 out]
            n156 = property on="Rev/Fwd" class="Clust (strict)"("Visible"=w307) -> ()  [unwired: 2 in, 2 out]
            n157 = property on="On/Off" class="Bool (strict)"("Visible"=w307) -> ()  [unwired: 2 in, 2 out]
            n158 = property on="Slider" class="Slide (strict)"("Visible"=w307) -> ()  [unwired: 2 in, 2 out]
          }
          frame "Motor", "PWM" {
            w313 = FALSE ("Visible")
            n159 = case shown="\"Motor\", Default" w312 {
              tunnel: [1.0 ("Value") -1.0 ("Value")] -> w311
              tunnel: [255.0 ("Value") 1.0 ("Value")] -> w310
              tunnel: [128.0 ("Value") 0.0 ("Value")] -> w309
              tunnel: [64.0 ("Value") 0.5 ("Value")] -> w308
              frame "PWM" {
              }
              frame "Motor", Default {
              }
            }
            n160 = property on="Motor" class="Clust (strict)"("Visible"=TRUE) -> ()  [unwired: 2 in, 2 out]
            n161 = property on="Value" class="Slide (strict)"("Value"=w309, "Scale.Minimum"=w311, "Scale.Maximum"=w310, "Scale.Increment"=w308) -> ()  [unwired: 2 in, 2 out]
            n162 = property on="On/Off" class="Bool (strict)"("Visible"=w313) -> ()  [unwired: 2 in, 2 out]
            n163 = property on="Slider" class="Slide (strict)"("Visible"=w313) -> ()  [unwired: 2 in, 2 out]
            n164 = property on="Ring" class="Ring (strict)"("Visible"=w313) -> ()  [unwired: 2 in, 2 out]
            n165 = property on="Rev/Fwd" class="Clust (strict)"("Visible"=w313) -> ()  [unwired: 2 in, 2 out]
          }
          frame "Servo" {
            w325 = FALSE ("Visible")
            n166 = call <vilib>:"NT Read Number.vi"("Name"=w327) -> ("Numeric"=w326:dbl)  [unwired: 9 in, 1 out]
            n167 = property on="Slider" class="Slide (strict)"("Visible"=TRUE, "Scale.Maximum"=170.0 ("Scale.Range:Maximum")) -> ()  [unwired: 2 in, 2 out]
            n168 = local write "Slider"(w326) -> ()
            n169 = property on="Motor" class="Clust (strict)"("Visible"=w325) -> ()  [unwired: 2 in, 2 out]
            n170 = property on="Rev/Fwd" class="Clust (strict)"("Visible"=w325) -> ()  [unwired: 2 in, 2 out]
            n171 = property on="On/Off" class="Bool (strict)"("Visible"=w325) -> ()  [unwired: 2 in, 2 out]
            n172 = property on="Ring" class="Ring (strict)"("Visible"=w325) -> ()  [unwired: 2 in, 2 out]
          }
          frame "Relay", "Solenoid" {
            w328 = FALSE ("Visible")
            n173 = property on="Motor" class="Clust (strict)"("Visible"=w328) -> ()  [unwired: 2 in, 2 out]
            n174 = property on="Slider" class="Slide (strict)"("Visible"=w328) -> ()  [unwired: 2 in, 2 out]
            n175 = Search and Replace String(input string=w329, search string="/Value  **", replace string="/Direction") -> (result string=w335:string)  [unwired: 5 in, 3 out]
            n176 = property on="Ring" class="Ring (strict)"("Visible"=w328) -> ()  [unwired: 2 in, 2 out]
            n177 = call <vilib>:"NT Read String.vi"("Name"=w335) -> ("String"=w333:string)  [unwired: 9 in, 1 out]
            n178 = Equal?(x="Both directions", y=w333) -> (x = y?=w331:bool)
            n179 = Not(x=w331) -> (.not. x?=w332:bool)
            n180 = property on="Rev/Fwd" class="Clust (strict)"("Visible"=w331) -> ()  [unwired: 2 in, 2 out]
            n181 = property on="On/Off" class="Bool (strict)"("Visible"=w332, "Caption.Text"=w330) -> ()  [unwired: 2 in, 2 out]
          }
          frame "Compressor", "Digital Out" {
            w338 = FALSE ("Visible")
            # "Get direction and finish"
            n182 = property on="Motor" class="Clust (strict)"("Visible"=w338) -> ()  [unwired: 2 in, 2 out]
            n183 = property on="Slider" class="Slide (strict)"("Visible"=w338) -> ()  [unwired: 2 in, 2 out]
            n184 = property on="Ring" class="Ring (strict)"("Visible"=w338) -> ()  [unwired: 2 in, 2 out]
            n185 = property on="On/Off" class="Bool (strict)"("Visible"=TRUE, "Caption.Text"=w339) -> ()  [unwired: 2 in, 2 out]
            n186 = property on="Rev/Fwd" class="Clust (strict)"("Visible"=FALSE) -> ()  [unwired: 2 in, 2 out]
          }
          frame "Camera" {
            n187 = call <vilib>:"Get Last Path Segment.vi"("String in"=w346) -> ("String out"=w347:string)  [unwired: 10 in]
            n188 = property on="On/Off" class="Bool (strict)"("Visible"=FALSE) -> ()  [unwired: 2 in, 2 out]
            n189 = property on="Motor" class="Clust (strict)"("Visible"=FALSE) -> ()  [unwired: 2 in, 2 out]
            n190 = property on="Rev/Fwd" class="Clust (strict)"("Visible"=FALSE) -> ()  [unwired: 2 in, 2 out]
            n191 = case shown="\"White Balance  **\"" w347 {
              tunnel: w346 -> [w353 w362 w371 w380 w389 _ w395]
              tunnel: w345 -> [w351 w359 w368 w377 w386 _ _]
              frame "Size  **" {
                n192 = Index Array(array=w351) -> (element=w350:cluster{string[]})  [unwired: 1 in]
                n193 = call <vilib>:"NT Read String.vi"("Name"=w353) -> ("String"=w352:string)  [unwired: 9 in, 1 out]
                n194 = Unbundle(w350) -> (w348:string[])
                n195 = Match First String(2:w348, 3:w352) -> (0:w349:i32)  [unwired: 1 out]
                n196 = property on="Ring" class="Ring (strict)"("Value"=w349, "Strings []"=w348) -> ()  [unwired: 2 in, 2 out]
                n197 = property on="Ring" class="Ring (strict)"("Visible"=TRUE) -> ()  [unwired: 2 in, 2 out]
                n198 = property on="Slider" class="Slide (strict)"("Visible"=FALSE) -> ()  [unwired: 2 in, 2 out]
              }
              frame "White Balance  **" {
                n199 = Index Array(array=w359, index=1) -> (element=w360:cluster{string[]})
                n200 = call <vilib>:"NT Read String.vi"("Name"=w362) -> ("String"=w361:string)  [unwired: 9 in, 1 out]
                n201 = Unbundle(w360) -> (w357:string[])
                n202 = Match First String(2:w357, 3:w361) -> (0:w356:i32)  [unwired: 1 out]
                n203 = property on="Ring" class="Ring (strict)"("Value"=w356, "Strings []"=w357) -> ()  [unwired: 2 in, 2 out]
                n204 = property on="Ring" class="Ring (strict)"("Visible"=TRUE) -> ()  [unwired: 2 in, 2 out]
                n205 = property on="Slider" class="Slide (strict)"("Visible"=FALSE) -> ()  [unwired: 2 in, 2 out]
              }
              frame "Exposure  **" {
                n206 = Index Array(array=w368, index=2) -> (element=w369:cluster{string[]})
                n207 = call <vilib>:"NT Read String.vi"("Name"=w371) -> ("String"=w370:string)  [unwired: 9 in, 1 out]
                n208 = Unbundle(w369) -> (w365:string[])
                n209 = Match First String(2:w365, 3:w370) -> (0:w366:i32)  [unwired: 1 out]
                n210 = property on="Ring" class="Ring (strict)"("Value"=w366, "Strings []"=w365) -> ()  [unwired: 2 in, 2 out]
                n211 = property on="Ring" class="Ring (strict)"("Visible"=TRUE) -> ()  [unwired: 2 in, 2 out]
                n212 = property on="Slider" class="Slide (strict)"("Visible"=FALSE) -> ()  [unwired: 2 in, 2 out]
              }
              frame "Exposure Priority  **" {
                n213 = Index Array(array=w377, index=3) -> (element=w378:cluster{string[]})
                n214 = call <vilib>:"NT Read String.vi"("Name"=w380) -> ("String"=w379:string)  [unwired: 9 in, 1 out]
                n215 = Unbundle(w378) -> (w374:string[])
                n216 = Match First String(2:w374, 3:w379) -> (0:w375:i32)  [unwired: 1 out]
                n217 = property on="Ring" class="Ring (strict)"("Value"=w375, "Strings []"=w374) -> ()  [unwired: 2 in, 2 out]
                n218 = property on="Ring" class="Ring (strict)"("Visible"=TRUE) -> ()  [unwired: 2 in, 2 out]
                n219 = property on="Slider" class="Slide (strict)"("Visible"=FALSE) -> ()  [unwired: 2 in, 2 out]
              }
              frame "Color Enable  **" {
                n220 = Index Array(array=w386, index=4) -> (element=w387:cluster{string[]})
                n221 = call <vilib>:"NT Read String.vi"("Name"=w389) -> ("String"=w388:string)  [unwired: 9 in, 1 out]
                n222 = Unbundle(w387) -> (w383:string[])
                n223 = Match First String(2:w383, 3:w388) -> (0:w384:i32)  [unwired: 1 out]
                n224 = property on="Ring" class="Ring (strict)"("Value"=w384, "Strings []"=w383) -> ()  [unwired: 2 in, 2 out]
                n225 = property on="Ring" class="Ring (strict)"("Visible"=TRUE) -> ()  [unwired: 2 in, 2 out]
                n226 = property on="Slider" class="Slide (strict)"("Visible"=FALSE) -> ()  [unwired: 2 in, 2 out]
              }
              frame Default {
                n227 = property on="Ring" class="Ring (strict)"("Visible"=FALSE) -> ()  [unwired: 2 in, 2 out]
                n228 = property on="Slider" class="Slide (strict)"("Visible"=FALSE) -> ()  [unwired: 2 in, 2 out]
              }
              frame "Brightness  **", "Color Level  **", "Compression  **", "FPS  **", "Sharpness  **" {
                n229 = call <vilib>:"NT Read Number.vi"("Name"=w395) -> ("Numeric"=w394:dbl)  [unwired: 9 in, 1 out]
                n230 = local write "Slider"(w394) -> ()
                n231 = property on="Slider" class="Slide (strict)"("Visible"=TRUE, "Scale.Maximum"=100.0 ("Scale.Range:Maximum")) -> ()  [unwired: 2 in, 2 out]
                n232 = property on="Ring" class="Ring (strict)"("Visible"=FALSE) -> ()  [unwired: 2 in, 2 out]
              }
            }
          }
        }
        n233 = property on="Progress" class="Clust (strict)"("Visible"=FALSE) -> ()  [unwired: 2 in, 2 out]
      }
      event "Test Name": Mouse Enter {
        # "Populate the ring with the list of tests"
        n234 = event-data() -> ()  [unwired: 1 in, 1 out]
        n235 = call <vilib>:"NT Read String Array.vi"("Name"="TestMode/TestList") -> ("String Array"=w402:string[])  [unwired: 9 in, 1 out]
        n236 = Build Array (concatenate)("Select the test to run...", w402) -> (w401:string[])
        n237 = property on="Test Name" class="Ring (strict)"("Strings []"=w401) -> ()  [unwired: 2 in, 2 out]
      }
      event "Test Name": Value Change {
        w404 = FALSE ("Visible")
        # "Tell the robot the test name to run"
        n238 = event-data() -> ("NewVal"=w408:u16)  [unwired: 1 in]
        n239 = property on="Test Name" class="Ring (strict)"() -> ("Strings []"=w409:string[])  [unwired: 2 in, 2 out]
        n240 = local write "Progress"(T7 {"Test Progress"=0, "Test Progress Text"=""} ("Progress")) -> ()
        n241 = Index Array(array=w409, index=w408) -> (element=w407:string)
        n242 = call <vilib>:"NT Write String.vi"("String"=w407, "Name"="TestMode/TestName") -> ()  [unwired: 9 in, 1 out]
        n243 = property on="Progress" class="Clust (strict)"("Visible"=TRUE) -> ()  [unwired: 2 in, 2 out]
        n244 = property on="Motor" class="Clust (strict)"("Visible"=w404) -> ()  [unwired: 2 in, 2 out]
        n245 = property on="Slider" class="Slide (strict)"("Visible"=w404) -> ()  [unwired: 2 in, 2 out]
        n246 = property on="On/Off" class="Bool (strict)"("Visible"=w404) -> ()  [unwired: 2 in, 2 out]
        n247 = property on="Rev/Fwd" class="Clust (strict)"("Visible"=w404) -> ()  [unwired: 2 in, 2 out]
        n248 = property on="Ring" class="Ring (strict)"("Visible"=w404) -> ()  [unwired: 2 in, 2 out]
      }
      event "Listbox": Double Click {
        n249 = event-data() -> ("PlatMods.Shift"=w412:bool, "Row"=w414:i32)  [unwired: 1 in]
        n250 = case shown="False" w412 {
          tunnel: w414 -> [w418 _]
          tunnel: 1 -> [w417 _]
          frame False {
            n251 = property on="Listbox" class="LstBox (strict)"() -> ("Item Symbols"=w416:i32[])  [unwired: 2 in, 2 out]
            n252 = Replace Array Subset(array=w416, new element=w417, index=w418) -> (w415:i32[])
            n253 = property on="Listbox" class="LstBox (strict)"("Item Symbols"=w415) -> ()  [unwired: 2 in, 2 out]
          }
          frame True {
            w419 = 0 ("Top Row")
            n254 = property on="Listbox" class="LstBox (strict)"() -> ("Number of Rows"=w421:u32)  [unwired: 2 in, 2 out]
            n255 = Initialize Array(0, w421) -> (w420:i32[])
            n256 = property on="Listbox" class="LstBox (strict)"("Top Row"=w419, "Value"=w419, "Item Symbols"=w420) -> ()  [unwired: 2 in, 2 out]
          }
        }
      }
      event "Listbox": Key Down {
        n257 = event-data() -> ("VKey"=w425:T22)  [unwired: 1 in]
        n258 = case shown="\"Left\", \"Right\"" w425 {
          selector: w425 -> [w430 _]
          tunnel: eventvkey."Left" ("VKey") -> [w428 _]
          frame "Left", "Right" {
            n259 = Equal?(x=w428, y=w430) -> (x = y?=w429:bool)
            n260 = Select(t=0, s=w429, f=1) -> (s? t:f=w431:i32)
            n261 = property on="Listbox" class="LstBox (strict)"() -> ("Item Symbols"=w434:i32[])  [unwired: 2 in, 2 out]
            n262 = Replace Array Subset(array=w434, new element=w431, index="Listbox") -> (w433:i32[])
            n263 = property on="Listbox" class="LstBox (strict)"("Item Symbols"=w433) -> ()  [unwired: 2 in, 2 out]
          }
          frame Default {
          }
        }
      }
      event "DB Camera Config": Value Change {
        n264 = event-data() -> ("NewVal"=w438:bool)  [unwired: 1 in]
        n265 = case shown="False" w438 {
          tunnel: w437 -> [w447 _]
          tunnel: [w440 w458] -> w436
          tunnel: w435 -> [w439 w458]
          frame False {
            w454 = "Camera"
            w457 = FALSE ("Visible")
            n266 = local read "Camera Settings"() -> (w446:T1)
            n267 = Index Array(array=w447) -> (element=w450:cluster{string[]})  [unwired: 1 in]
            n268 = Unbundle(w446) -> ("Frate Rate"=w445:i32, "Compression"=w444:i32, "Size"=w448:u16)
            n269 = Unbundle(w450) -> (w449:string[])
            n270 = Index Array(array=w449, index=w448) -> (element=w443:string)
            n271 = call-poly <vilib>:"Write Key.vi"("section"=w454, "value"=w443, "key"="Size", "refnum"=w439) -> ("refnum out"=w456:T21)  [unwired: 2 in, 5 out]
            n272 = call-poly <vilib>:"Write Key.vi"("section"=w454, "value"=w445, "key"="FrameRate", "refnum"=w456) -> ("refnum out"=w455:T21)  [unwired: 1 in, 6 out]
            n273 = property on="Camera Settings" class="Clust (strict)"("Visible"=w457) -> ()  [unwired: 2 in, 2 out]
            n274 = local write "DB Camera Config"(w457) -> ()
            n275 = call-poly <vilib>:"Write Key.vi"("section"=w454, "value"=w444, "key"="Compression", "refnum"=w455) -> ("refnum out"=w441:T21)  [unwired: 1 in, 6 out]
            n276 = call <vilib>:"Close Config Data.vi"("refnum"=w441) -> ("file path"=w442:path)  [unwired: 2 in, 8 out]
            n277 = call <vilib>:"Open Config Data.vi"("configuration file path"=w442) -> ("refnum"=w440:T21)  [unwired: 8 in, 2 out]
          }
          frame True {
            n278 = property on="Camera Settings" class="Clust (strict)"("Visible"=TRUE) -> ()  [unwired: 2 in, 2 out]
          }
        }
      }
      event "Camera Settings": Value Change {
        n279 = event-data() -> ("NewVal"=w471:T1)  [unwired: 1 in]
        n280 = Index Array(array=w467) -> (element=w466:cluster{string[]})  [unwired: 1 in]
        n281 = Unbundle(w471) -> ("Frate Rate"=w462:i32, "Compression"=w461:i32, "Size"=w464:u16)
        n282 = Unbundle(w466) -> (w465:string[])
        n283 = Index Array(array=w465, index=w464) -> (element=w463:string)
        n284 = Format Into String(format string="%s   %dfps   %d%%", w463, w462, w461) -> (resulting string=w468:string)  [unwired: 2 in, 1 out]
        n285 = Build Array(w468) -> (w469:string[])
        n286 = property on="DB Camera Config" class="Bool (strict)"("Strings [4]"=w469) -> ()  [unwired: 2 in, 2 out]
      }
      event "Motor.Enable": Value Change {
        n287 = event-data() -> ("NewVal"=w477:bool)  [unwired: 1 in]
        n288 = Unbundle("Motor") -> ("Value"=w476:dbl)  [unwired: 1 out]
        n289 = Select(t=w476, s=w477, f=0.0) -> (s? t:f=w474:dbl)
        n290 = call <vilib>:"NT Write Number.vi"("Numeric"=w474, "Name"=w473) -> ()  [unwired: 9 in, 1 out]
      }
      event "Slider": Value Change {
        n291 = event-data() -> ("NewVal"=w480:dbl)  [unwired: 1 in]
        n292 = call <vilib>:"NT Write Number.vi"("Numeric"=w480, "Name"=w481) -> ()  [unwired: 9 in, 1 out]
      }
      event "On/Off": Value Change {
        n293 = event-data() -> ("NewVal"=w485:bool)  [unwired: 1 in]
        n294 = Boolean To (0,1)(Boolean=w485) -> (0, 1=w484:i16)
        n295 = call <vilib>:"NT Write Number.vi"("Numeric"=w484, "Name"=w483) -> ()  [unwired: 9 in, 1 out]
      }
      event "Rev/Fwd": Value Change {
        n296 = event-data() -> ("NewVal.Forward"=w493:bool, "NewVal.Reverse"=w492:bool)  [unwired: 1 in]
        n297 = Boolean To (0,1)(Boolean=w493) -> (0, 1=w489:i16)
        n298 = Boolean To (0,1)(Boolean=w492) -> (0, 1=w491:i16)
        n299 = Negate(x=w491) -> (-x=w490:i16)
        n300 = Add(x=w489, y=w490) -> (x+y=w488:i16)
        n301 = call <vilib>:"NT Write Number.vi"("Numeric"=w488, "Name"=w487) -> ()  [unwired: 9 in, 1 out]
      }
      event "Ring": Value Change {
        n302 = event-data() -> ("NewVal"=w497:u16)  [unwired: 1 in]
        n303 = property on="Ring" class="Ring (strict)"() -> ("Strings []"=w498:string[])  [unwired: 2 in, 2 out]
        n304 = Index Array(array=w498, index=w497) -> (element=w496:string)
        n305 = call <vilib>:"NT Write String.vi"("String"=w496, "Name"=w495) -> ()  [unwired: 9 in, 1 out]
      }
    }
  }
  n306 = Index Array(array=w17) -> (element=w18:cluster{string[]})  [unwired: 1 in]
  n307 = disable-structure shown="Disabled" {
    frame Disabled {
      # "Blink at 6 Hz"
      n308 = Tick Count (ms)() -> (millisecond timer value=w499:u32)
      n309 = Divide(x=1000, y=12) -> (x/y=w502:dbl)
      n310 = Divide(x=w499, y=w502) -> (x/y=w504:dbl)
      n311 = Round Toward -Infinity(1:w504) -> (0:w505:dbl)
      n312 = Quotient & Remainder(x=w505, y=2) -> (x-y*floor(x/y)=w506:dbl)  [unwired: 1 out]
      n313 = Equal?(x=w506, y=0.0) -> (x = y?=w508:bool)
    }
    frame Enabled {
    }
  }
  n314 = Unbundle(w18) -> (w16:string[])
  n315 = Match First String(2:w16, 3:w15) -> (0:w14:i32)  [unwired: 1 out]
  n316 = Bundle("value"=w20, "value"=w19, "index"=w14) -> (w8:cluster{"value":i32, "value":i32, "index":i32})  [unwired: 1 out]
  n317 = property on="On/Off" class="Bool (strict)"("Visible"=w31) -> ()  [unwired: 2 in, 2 out]
  n318 = property on="Motor" class="Clust (strict)"("Visible"=w31) -> ()  [unwired: 2 in, 2 out]
  n319 = property on="Progress" class="Clust (strict)"("Visible"=w31) -> ()  [unwired: 2 in, 2 out]
  n320 = property on="Ring" class="Ring (strict)"("Visible"=w31) -> ()  [unwired: 2 in, 2 out]
  n321 = property on="Camera Settings" class="Clust (strict)"("Val(Sgnl)"=w8) -> ()  [unwired: 2 in, 2 out]
  n322 = property on="Rev/Fwd" class="Clust (strict)"("Visible"=w31) -> ()  [unwired: 2 in, 2 out]
  n323 = property on="Camera Settings" class="Clust (strict)"("Visible"=w31) -> ()  [unwired: 2 in, 2 out]
  n324 = local write "DB Camera Config"(w31) -> ()
  "Dashboard Code Verzion" <- "Vision Dash 1.5 DEV" ("Dashboard Code Verzion")
